vi "Get Process Memory Info x64.vi"(8 "error in (no error)":errorcluster) -> (0 "error out":errorcluster, 2 "Memory Usage by Labview(GB)":dbl, 3 "ppsmemCounters":T1)   [LabVIEW 2018]
uses:
  kernel32.dll
  Psapi.dll
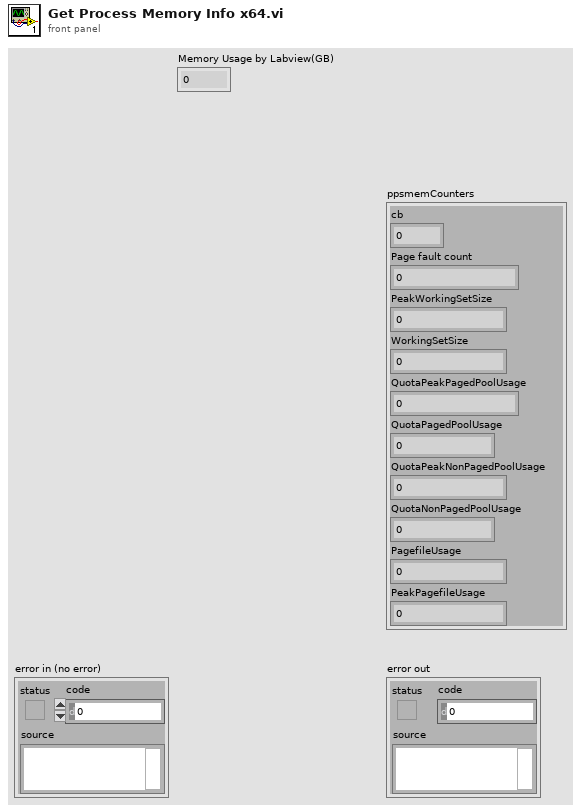
[diagram p1: front panel]
types:
  T1 = cluster{"cb":u32, "Page fault count":u32, "PeakWorkingSetSize":u64, "WorkingSetSize":u64, "QuotaPeakPagedPoolUsage":u64, "QuotaPagedPoolUsage":u64, "QuotaPeakNonPagedPoolUsage":u64, "QuotaNonPagedPoolUsage":u64, "PagefileUsage":u64, "PeakPagefileUsage":u64}
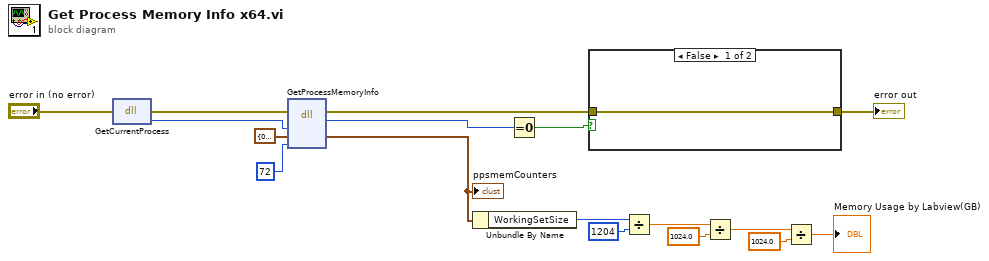
[diagram p0: block diagram]
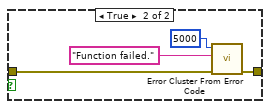
[diagram p2: hidden frame]
diagram:
  n1 = dll-call lib="kernel32.dll" fn="GetCurrentProcess"(error in="error in (no error)") -> (error out=w16:errorcluster, "return type"=w17:u64)  [unwired: 2 in, 1 out]
  n2 = dll-call lib="Psapi.dll" fn="GetProcessMemoryInfo"(error in=w16, "Process"=w17, "ppsmemCounters"=T1 {"cb"=0, "Page fault count"=0, "PeakWorkingSetSize"=0, "WorkingSetSize"=0, "QuotaPeakPagedPoolUsage"=0, "QuotaPagedPoolUsage"=0, "QuotaPeakNonPagedPoolUsage"=0, "QuotaNonPagedPoolUsage"=0, "PagefileUsage"=0, "PeakPagefileUsage"=0} ("Cluster"), "cb"=u32 72) -> (error out=w9:errorcluster, "return type"=w13:i32, "ppsmemCounters"=w8:T1)  [unwired: 4 in, 1 out]
  "ppsmemCounters" <- w8
  n3 = Unbundle By Name(w8) -> ("WorkingSetSize"=w7:u64)
  n4 = Equal To 0?(x=w13) -> (x = 0?=w12:bool)
  n5 = case shown="False" w12 {
    tunnel: w9 -> [w18 w22]
    tunnel: [w18 w21] -> w11
    frame False {
    }
    frame True {
      n6 = call <vilib>:"Error Cluster From Error Code.vi"("error in (no error)"=w22, "error message (\"\")"="Function failed." ("error message (\"\")"), "error code (0)"=5000) -> ("error out"=w21:errorcluster)  [unwired: 6 in]
    }
  }
  "error out" <- w11
  n7 = Divide(x=w7, y=u64 1204) -> (x/y=w6:dbl)
  n8 = Divide(x=w6, y=1024.0) -> (x/y=w5:dbl)
  n9 = Divide(x=w5, y=1024.0) -> (x/y=→"Memory Usage by Labview(GB)":dbl)
